vi "GetParam.vi"(8 "error in (no error)":errorcluster caption="entrée d'erreur (pas d'erreur)", 11 "MissingIndicator.lvclass":refnum<class "MissingIndicator.lvclass">) -> (0 "error out":errorcluster caption="sortie d'erreur", 2 "MissingIndicator":T1={"missing_values"="nan", "features"="None", "sparse"="None", "error_on_new"=TRUE}, 3 "MissingIndicator.lvclass":refnum<class "MissingIndicator.lvclass">)   [LabVIEW 2020, in "MissingIndicator.lvclass"]
doc: "Get Parameters"
uses:
  MissingIndicator.lvclass
  MissingIndicator.lvclass/MissingIndicator.ctl
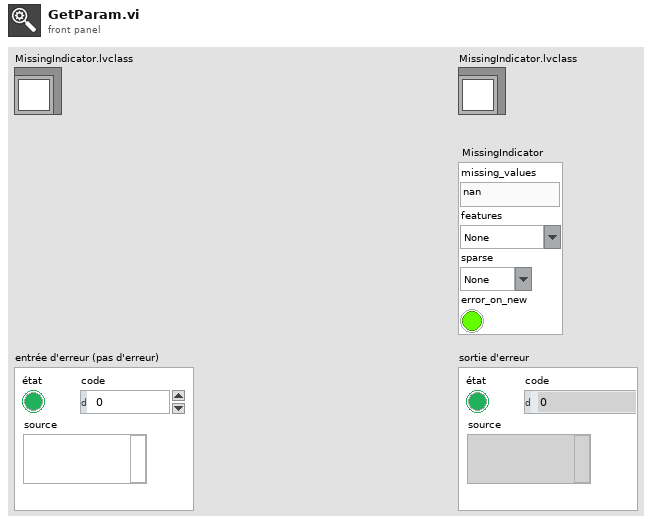
[diagram p1: front panel]
types:
  T1 = cluster{"missing_values":string, "features":string, "sparse":string, "error_on_new":bool}
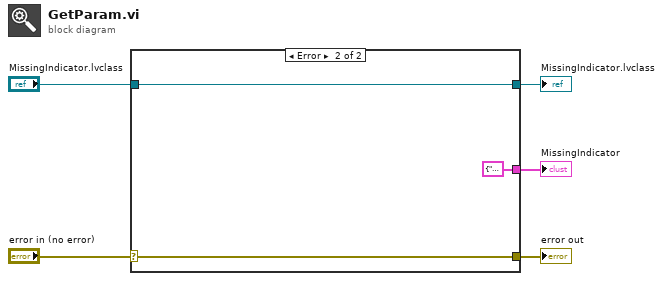
[diagram p0: block diagram]
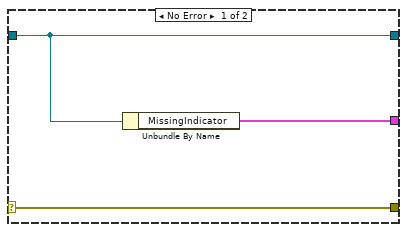
[diagram p2: hidden frame]
diagram:
  n1 = case shown="Error" "error in (no error)" {
    selector: "error in (no error)" -> [w8 w10]
    tunnel: [w8 w10] -> w4
    tunnel: [w7 w11] -> w2
    tunnel: "MissingIndicator.lvclass" -> [w7 w11]
    tunnel: [w6 T1 {"missing_values"="", "features"="", "sparse"="", "error_on_new"=FALSE} ("MissingIndicator")] -> w1
    frame No Error {
      n2 = Unbundle By Name(w7) -> ("MissingIndicator"=w6:T1)
    }
    frame Error {
    }
  }
  "error out" <- w4
  "MissingIndicator.lvclass" <- w2
  "MissingIndicator" <- w1
